vi "LCA Write Pos Marker Mode.vi"(8 "error in (no error)":errorcluster caption="Fehler (Eingang, kein Fehler)", 10 "Position Marker Mode Mode":u8, 11 "Axis Handle":i64) -> (0 "error out":errorcluster caption="Fehler (Ausgang)")   [LabVIEW 2021, in "labbCAN_MotionControl_API.lvlib"]
doc: "LCA_Func long __stdcall LCA_WritePosMarkerMode(dev_hdl hAxis,\n unsigned char Mode);"
uses:
  labbCAN_MotionControl_API.lvlib
  labbCAN_MotionControl_API.dll
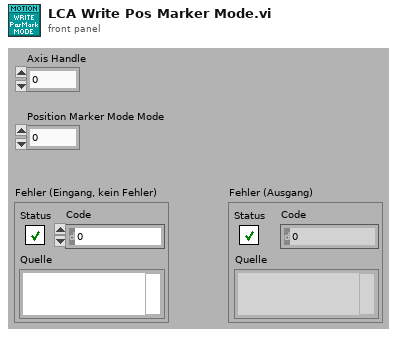
[diagram p1: front panel]
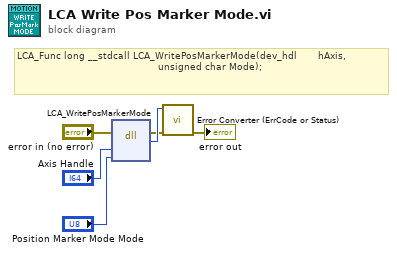
[diagram p0: block diagram]
diagram:
  # "LCA_Func long __stdcall LCA_WritePosMarkerMode(dev_hdl       hAxis,\n                                               unsigned char Mode);"
  n1 = dll-call lib="C:/Users/olaja/AppData/Local/CETONI_SDK/labbCAN_MotionControl_API.*" fn="LCA_WritePosMarkerMode"(error in="error in (no error)", "hAxis"="Axis Handle", "Mode"="Position Marker Mode Mode") -> (error out=w2:errorcluster, "Rückgabetyp"=w6:i32)  [unwired: 4 in, 1 out]
  n2 = call "Error Converter (ErrCode or Status).vi"("error in (no error)"=w2, "error code"=w6) -> ("error out"=→"error out":errorcluster)  [unwired: 9 in]
